vi "Execute Command.vi"(8 "error in (no error)":errorcluster, 10 "Command In":refnum<class "Command.lvclass">, 11 "Executing in":refnum<class "Executing.lvclass">) -> (0 "error out":errorcluster, 3 "Executing out":refnum<class "Executing.lvclass">)   [LabVIEW 2013, in "Command Processor.lvlib" / "Executing.lvclass"]
uses:
  Executing.lvclass
  Command/Command.lvclass
  Command Processor.lvclass
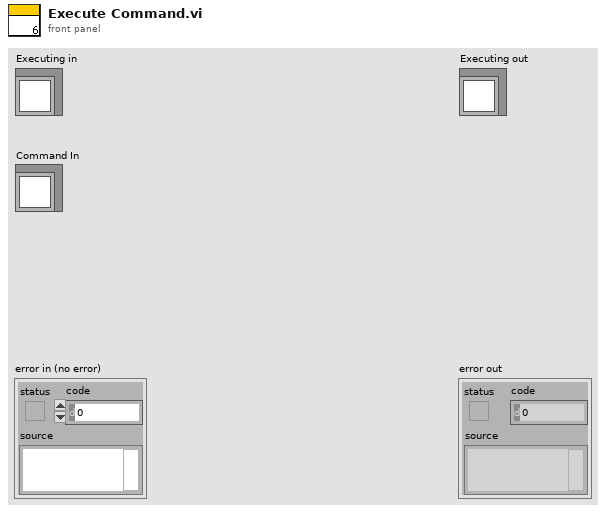
[diagram p1: front panel]
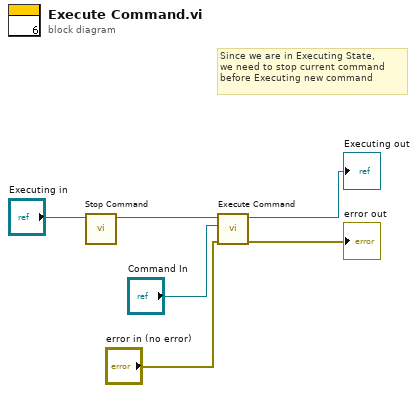
[diagram p0: block diagram]
diagram:
  # "Since we are in Executing State,\nwe need to stop current command \nbefore Executing new command"
  n1 = call-dynamic "Stop Command.vi"("Command Processor in"="Executing in") -> ("Command Processor out"=w1:refnum<class "Executing.lvclass">)  [unwired: 9 in, 1 out]
  n2 = call-parent "Execute Command.vi"("error in (no error)"="error in (no error)", "Command In"="Command In", "Command Processor in"=w1) -> ("error out"=→"error out":errorcluster, "Command Processor out"=→"Executing out":refnum<class "Executing.lvclass">)  [unwired: 7 in]
